vi "Actuators Startup.vi"() -> (3 "IO Cluster OUT":T1)   [LabVIEW 2019]
uses:
  Actuators IO Cluster.ctl
  <vilib>/FPGAPlugInAG/myRIO-1900/niLvFpga_Open_myRIO-1900.vi
  <vilib>/rvi/interface/common/dynamic/niFpgaDynamicAddResources.vi
  <vilib>/Utility/error.llb/Error Cluster From Error Code.vi
  <vilib>/rvi/errors/niLvFpgaAdjustHostInterfaceError.vi
  <vilib>/rvi/interface/nirviOpenFPGA/nirviOpenFPGA.xnode
  QAB Actuators FPGA.vi
  <vilib>/rvi/interface/nirviReadWriteControl/nirviReadWriteControl.xnode
  NiFpgaLv.dll
  <vilib>/rvi/interface/Simulation/niFpgaSimulationCallBeginRW.vi
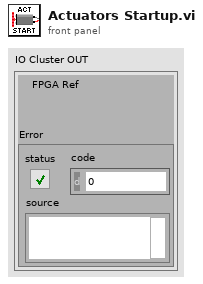
[diagram p1: front panel]
types:
  T1 = typedef "Actuators IO Cluster.ctl" = cluster{"Error":errorcluster, "FPGA Ref":refnum<k20>}
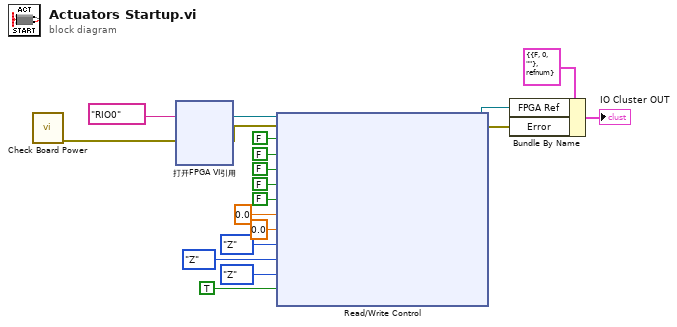
[diagram p0: block diagram]
diagram:
  n1 = call "Check Board Power.vi"() -> ("Error Out"=w1:errorcluster)  [unwired: 11 in]
  n2 = xnode "打开FPGA VI引用"("错误输入"=w1, "资源名称"=tag "RIO0" ("resource name")) -> ("FPGA VI引用输出"=w6:refnum<k20>, "错误输出"=w2:errorcluster)
  n3 = xnode "Read/Write Control"("FPGA VI引用输入"=w6, "错误输入"=w2, "Microstep Enable"=FALSE, "Stepper Control 1"=FALSE, "Stepper Control 2"=FALSE, "Stepper Control 3"=FALSE, "Stepper Control 4"=FALSE, "DC Linear Amplifier Value (+/-10)"=sgl 0.0, "DC Motor PWM (0-1)"=sgl 0.0, "BLDC Drive Phase A"=enum16{"H", "L", "Z"}."Z", "BLDC Drive Phase B"=enum16{"H", "L", "Z"}."Z", "BLDC Drive Phase C"=enum16{"H", "L", "Z"}."Z", "LED Status"=TRUE ("LED DC Motor")) -> ("FPGA VI引用输出"=w5:refnum<k20>, "错误输出"=w4:errorcluster)
  n4 = Bundle By Name(cluster=T1 {"Error"={"status"=FALSE, "code"=0, "source"=""}, "FPGA Ref"=refnum} ("Cluster"), "FPGA Ref"=w5, "Error"=w4) -> (→"IO Cluster OUT":T1)
